vi "Datos_to_TXT2.vi"(0 "Array":dbl[][](array[numeric]), 5 "Array 2":dbl[][](array[numeric]), 7 "Path":path, 9 "String":string, 11 "error in (no error)":errorcluster) -> (4 "spreadsheet string":string)   [LabVIEW 2019]
panel:
  out "output array":string[][](array[string])
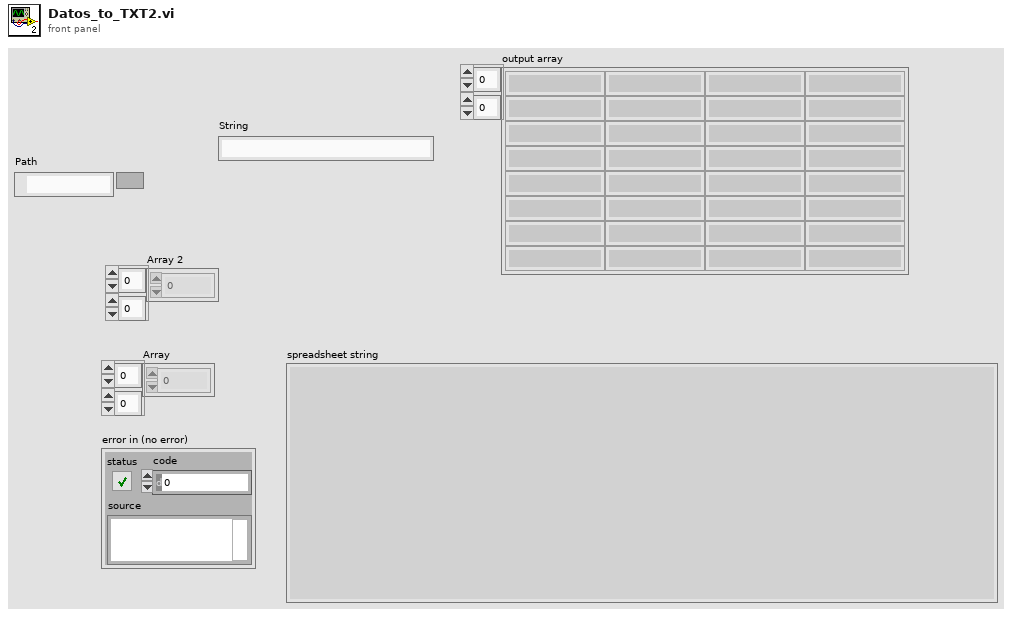
[diagram p1: front panel]
types:
  T1 = enum16{"open", "replace", "create", "open or create", "replace or create", "replace or create with confirmation"}
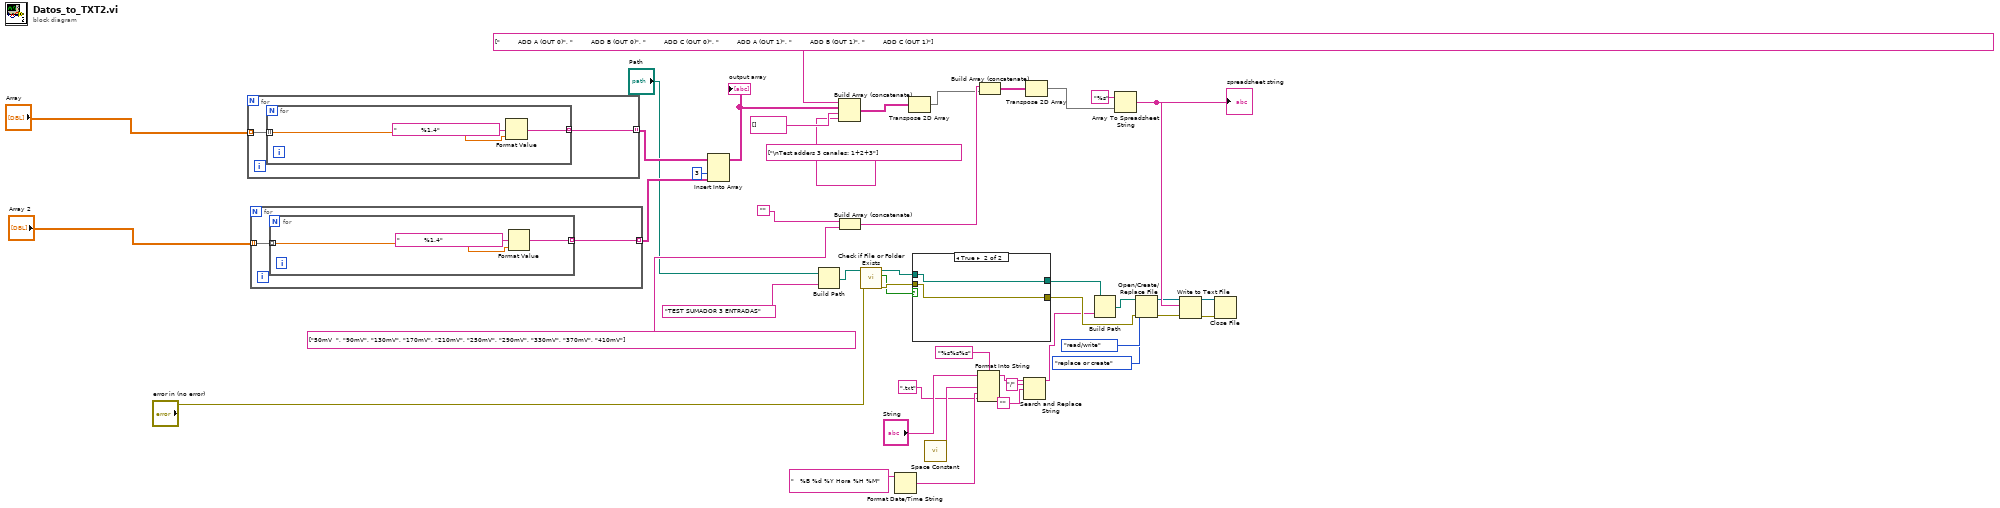
[diagram p0: block diagram]
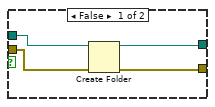
[diagram p2: hidden frame]
diagram:
  n1 = for {
    tunnel: "Array" -> [w46] mode=indexing
    tunnel: [w45] -> w16 mode=indexing
    n2 = for {
      tunnel: w46 -> [w48] mode=indexing
      tunnel: [w47] -> w45 mode=indexing
      n3 = Format Value(format string="            %1.4", value (0)=w48) -> (output string=w47:string)  [unwired: 1 in]
    }
  }
  n4 = for {
    tunnel: "Array 2" -> [w51] mode=indexing
    tunnel: [w50] -> w15 mode=indexing
    n5 = for {
      tunnel: w51 -> [w53] mode=indexing
      tunnel: [w52] -> w50 mode=indexing
      n6 = Format Value(format string="            %1.4", value (0)=w53) -> (output string=w52:string)  [unwired: 1 in]
    }
  }
  n7 = Insert Into Array(array=w16, index (col)=3 ("disabled index (col)"), new element=w15) -> (w13:string[][])  [unwired: 1 in]
  "output array" <- w13
  n8 = Build Path(base path="Path", name or relative path="TEST SUMADOR 3 ENTRADAS") -> (appended path=w29:path)
  n9 = Build Array (concatenate)(string[] ["         ADD A (OUT 0)", "         ADD B (OUT 0)", "         ADD C (OUT 0)", "         ADD A (OUT 1)", "         ADD B (OUT 1)", "         ADD C (OUT 1)"], w13, string[] [] ("array"), string[] ["\nTest adders 3 canales: 1+2+3"] ("element")) -> (w24:string[][])
  n10 = Build Array (concatenate)("", string[] ["50mV  ", "90mV", "130mV", "170mV", "210mV", "250mV", "290mV", "330mV", "370mV", "410mV"]) -> (w23:string[])
  n11 = call <vilib>:"Check if File or Folder Exists.vi"("error in (no error)"="error in (no error)", "path"=w29) -> ("error out"=w33:errorcluster, "file or folder exists?"=w31:bool, "dup path"=w32:path)  [unwired: 7 in]
  n12 = Format Date/Time String(time format string (%c)="   %B %d %Y Hora %H %M") -> (date/time string=w2:string)  [unwired: 2 in]
  n13 = Transpose 2D Array(2D array=w24) -> (transposed array=w22:string[][])
  n14 = case shown="True" w31 {
    tunnel: w32 -> [w57 w60]
    tunnel: w33 -> [w58 w59]
    tunnel: [w55 w59] -> w43
    tunnel: [w56 w60] -> w34
    frame False {
      n15 = Create Folder(path (use dialog)=w57, error in=w58) -> (created path=w56:path, error out=w55:errorcluster)  [unwired: 1 in, 1 out]
    }
    frame True {
    }
  }
  n16 = call <vilib>:"Space Constant.vi"() -> ("String"=w3:string)
  n17 = Format Into String(format string="%s%s%s", initial string="String", w3, w2, ".txt" ("input 2")) -> (resulting string=w8:string)  [unwired: 1 in, 1 out]
  n18 = Build Array (concatenate)(w23, w22) -> (w21:string[][])
  n19 = Search and Replace String(input string=w8, search string="/", replace string="") -> (result string=w5:string)  [unwired: 5 in, 3 out]
  n20 = Transpose 2D Array(2D array=w21) -> (transposed array=w20:string[][])
  n21 = Build Path(base path=w34, name or relative path=w5) -> (appended path=w36:path)
  n22 = Array To Spreadsheet String(array=w20, 3:"%s" ("format string")) -> (spreadsheet string=w44:string)  [unwired: 1 in]
  "spreadsheet string" <- w44
  n23 = Open/Create/Replace File(file path (use dialog)=w36, error in=w43, operation (0:open)=T1."replace or create", access (0:read/write)=enum16{"read/write", "read-only", "write-only"}."read/write") -> (refnum out=w39:refnum<file>, error out=w40:errorcluster)  [unwired: 2 in, 1 out]
  n24 = Write to Text File(file (use dialog)=w39, text=w44, error in=w40) -> (refnum out=w42:refnum<file>, error out=w41:errorcluster)  [unwired: 1 in, 1 out]
  n25 = Close File(refnum=w42, error in=w41) -> ()  [unwired: 2 out]
